vi "panelUpdate.vi"(8 "error in (no error)":errorcluster, 10 "Defer Panel Updates":bool, 11 "QControl_Graph in":refnum<class "QControl_Graph.lvclass">) -> (0 "error out":errorcluster, 3 "QControl_Graph out":refnum<class "QControl_Graph.lvclass">)   [LabVIEW 2017, in "QControl_Graph.lvclass"]
uses:
  QControl_Graph.lvclass
  C:/Program Files (x86)/National Instruments/LabVIEW 2017/vi.lib/QSI/QControls/QControl Classes/Generic/Generic.lvclass
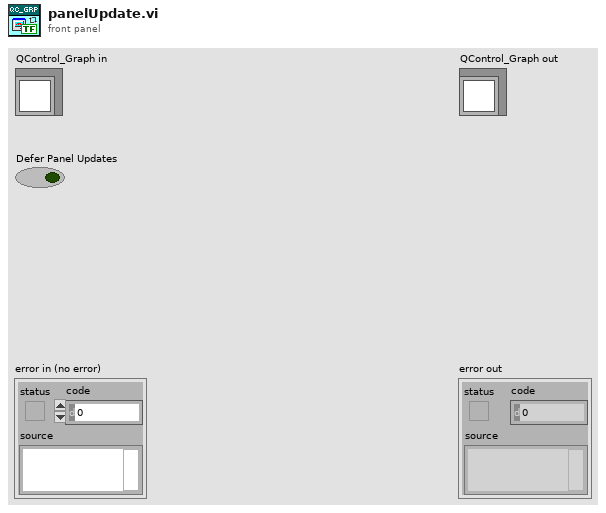
[diagram p1: front panel]
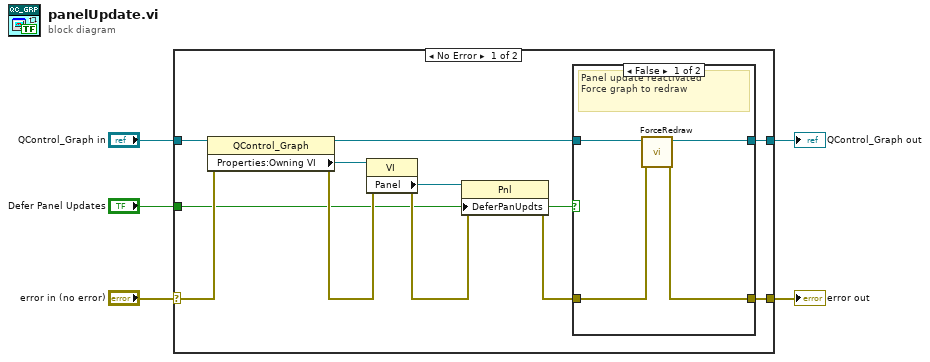
[diagram p0: block diagram]
diagram:
  n1 = case shown="No Error" "error in (no error)" {
    selector: "error in (no error)" -> [w13 w24]
    tunnel: [w7 w24] -> w4
    tunnel: [w9 w23] -> w2
    tunnel: "QControl_Graph in" -> [w16 w23]
    tunnel: "Defer Panel Updates" -> [w6 _]
    frame No Error {
      n2 = property class="QControl_Graph"(reference=w16, error in=w13) -> (reference out=w10:refnum<class "QControl_Graph.lvclass">, error out=w12:errorcluster, "Properties:Owning VI"=w15:refnum<vi>)
      n3 = property class="VI"(reference=w15, error in=w12) -> (error out=w11:errorcluster, "Panel"=w14:refnum<vi>)  [unwired: 1 out]
      n4 = property class="Pnl"(reference=w14, error in=w11, "DeferPanUpdts"=w6) -> (error out=w8:errorcluster)  [unwired: 1 out]
      n5 = case shown="False" w6 {
        tunnel: w10 -> [w20 w22]
        tunnel: [w19 w22] -> w9
        tunnel: w8 -> [w18 w21]
        tunnel: [w17 w21] -> w7
        frame False {
          # "Panel update reactivated \nForce graph to redraw"
          n6 = call-dynamic "ForceRedraw.vi"("error in (no error)"=w18, "GraphChart in"=w20) -> ("error out"=w17:errorcluster, "GraphChart out"=w19:refnum<class "QControl_Graph.lvclass">)  [unwired: 8 in]
        }
        frame True {
          # "Panel update deferred"
        }
      }
    }
    frame Error {
    }
  }
  "error out" <- w4
  "QControl_Graph out" <- w2
